vi "Close.vi"(8 "error in":errorcluster, 11 "UserEventHandler in":refnum<class "UserEventHandler.lvclass">) -> (0 "error out":errorcluster, 3 "UserEventHandler out":refnum<class "UserEventHandler.lvclass">)   [LabVIEW 2016, in "hse-logger.lvlib" / "UserEventHandler.lvclass"]
doc: "Destroys the user event. This method should be called when the ``Logger`` gets closed or the handler is removed from the ``Logger``."
uses:
  UserEventHandler.lvclass
  UserEventHandler.lvclass/UserEventHandler.ctl
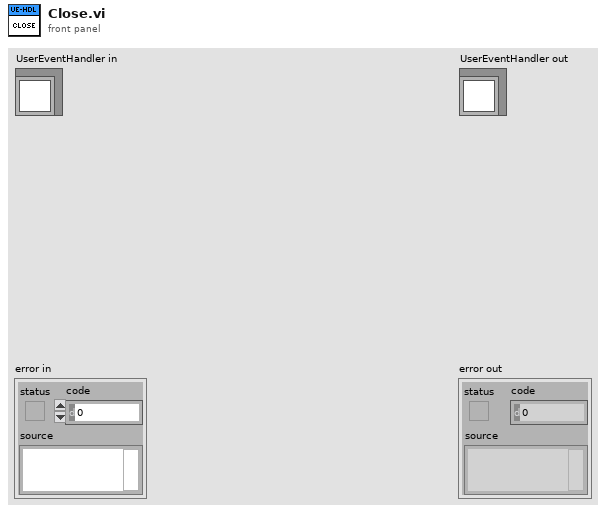
[diagram p1: front panel]
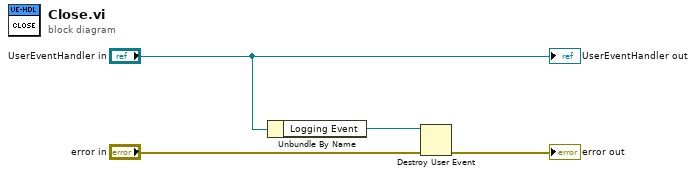
[diagram p0: block diagram]
diagram:
  n1 = Unbundle By Name("UserEventHandler in") -> ("Logging Event"=w1:refnum<user-event>)
  n2 = Destroy User Event(user event=w1, error in="error in") -> (error out=→"error out":errorcluster)
  "UserEventHandler out" <- "UserEventHandler in"
